vi "客户端校验.vi"() -> ()   [LabVIEW 2014]
panel:
  in  "退出":bool
  in  "生成":bool
  in  "license":string
  out "机器码":string
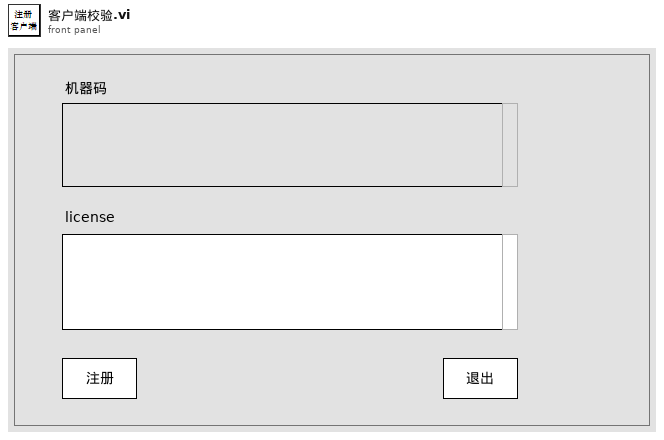
[diagram p1: front panel]
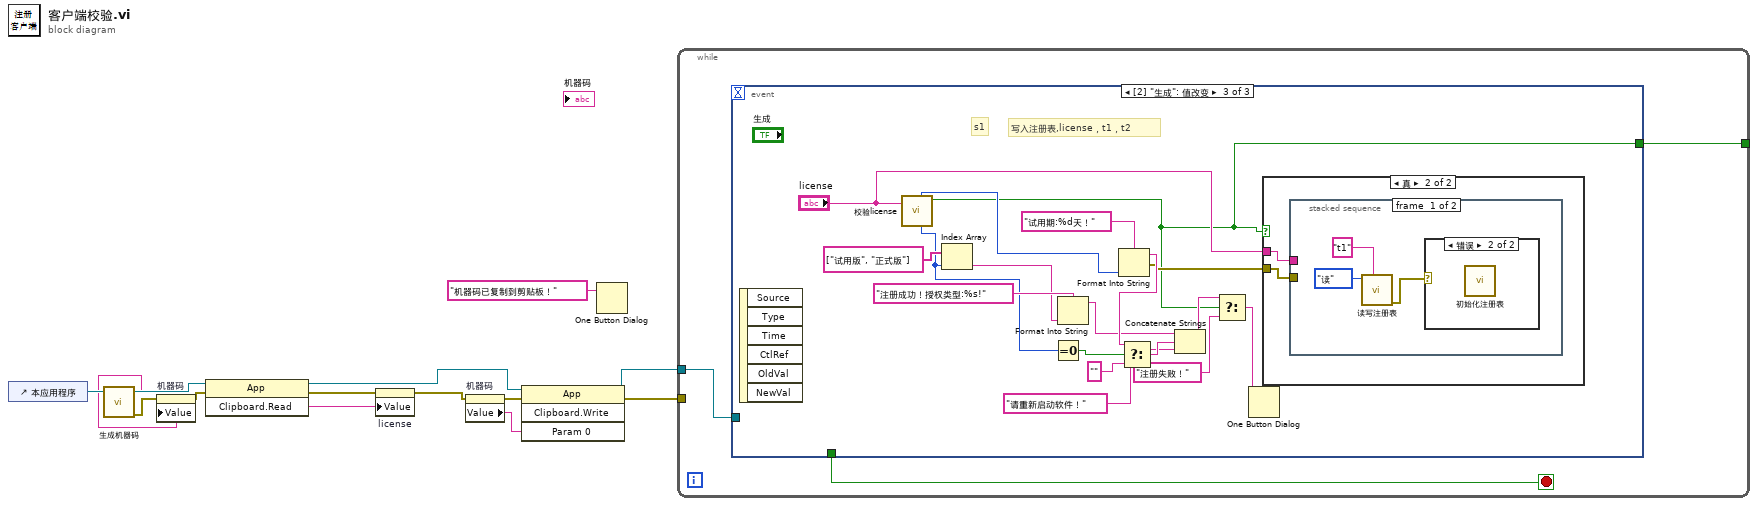
[diagram p0: block diagram]
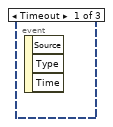
[diagram p2: hidden frame]
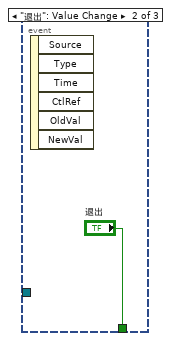
[diagram p3: hidden frame]
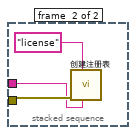
[diagram p6: hidden frame]
diagram:
  n1 = control-ref of="本应用程序"() -> (w13:refnum<vi>)
  n2 = call "生成机器码.vi"() -> ("error out"=w3:errorcluster, "机器码"=w1:string)  [unwired: 10 in]
  n3 = property on="机器码" class="Str"(error in=w3, "Value"=w1) -> (error out=w2:errorcluster)  [unwired: 1 in, 1 out]
  n4 = invoke class="App" method="Clipboard.Read"(reference=w13, error in=w2) -> (reference out=w9:refnum<vi>, error out=w12:errorcluster, "Read Clipbrd"=w11:string)  [unwired: 1 in]
  n5 = property on="license" class="Str"(error in=w12, "Value"=w11) -> (error out=w6:errorcluster)  [unwired: 1 in, 1 out]
  n6 = property on="机器码" class="Str"(error in=w6) -> (error out=w5:errorcluster, "Value"=w4:string)  [unwired: 1 in, 1 out]
  n7 = invoke class="App" method="Clipboard.Write"(reference=w9, error in=w5, "Param 0"=w4) -> (reference out=w8:refnum<vi>, error out=w7:errorcluster)  [unwired: 1 in, 2 out]
  n8 = One Button Dialog(message="机器码已复制到剪贴板！" ("消息")) -> ()  [unwired: 1 in, 1 out]
  n9 = while {
    tunnel: w8 -> [w16]
    tunnel: w7 -> [_]
    tunnel: [w14] -> _
    stop <- w15 stop-if-true
    n10 = event shown="[2] \"生成\": 值改变" {
      selector: _ -> [_ _ _]
      dyn-events: _ -> [_ _ _]
      timeout: _ -> [_ _ _]
      tunnel: w16 -> [_ _ _]
      tunnel: [_ "退出" _] -> w15
      tunnel: [_ _ w19] -> w14
      event Timeout {
        n11 = event-data() -> ()  [unwired: 1 in, 3 out]
      }
      event "退出": Value Change {
        n12 = event-data() -> ()  [unwired: 1 in, 6 out]
      }
      event "生成": Value Change {
        # "写入注册表,license，t1，t2"
        # "s1"
        n13 = event-data() -> ()  [unwired: 1 in, 6 out]
        n14 = call "校验license.vi"("license"="license") -> ("license正确"=w19:bool, "授权类型"=w30:i32, "T"=w31:u32)  [unwired: 7 in, 1 out]
        n15 = Index Array(array=string[] ["试用版", "正式版"] ("字符串[]"), index=w30) -> (element=w33:string)
        n16 = Equal To 0?(x=w30) -> (x = 0?=w29:bool)
        n17 = Format Into String(format string="注册成功！授权类型:%s!" ("格式字符串"), w33) -> (resulting string=w26:string)  [unwired: 2 in, 1 out]
        n18 = Format Into String(format string="试用期:%d天！" ("格式字符串"), w31) -> (resulting string=w28:string, error out=w21:errorcluster)  [unwired: 2 in]
        n19 = Select(t=w28, s=w29, f="") -> (s? t:f=w25:string)
        n20 = Concatenate Strings(w26, w25, "请重新启动软件！" ("字符串")) -> (w24:string)
        n21 = Select(t=w24, s=w19, f="注册失败！") -> (s? t:f=w22:string)
        n22 = One Button Dialog(message=w22) -> ()  [unwired: 1 in, 1 out]
        n23 = case shown="真" w19 {
          tunnel: w21 -> [_ w37]
          tunnel: "license" -> [_ w36]
          frame False {
          }
          frame True {
            n24 = stacked-sequence {
              tunnel: w37 -> [_ w43]
              tunnel: w36 -> [_ w41]
              frame #0 {
                n25 = call "读写注册表.vi"("键名称"="t1", "读/写"=enum16{"读", "写"}."读") -> ("error out"=w38:errorcluster)  [unwired: 8 in, 1 out]
                n26 = case shown="错误" w38 {
                  frame No Error {
                  }
                  frame Error {
                    n27 = call "初始化注册表.vi"() -> ()  [unwired: 11 in, 1 out]
                  }
                }
              }
              frame #1 {
                n28 = call "创建注册表.vi"("写入内容"=w41, "键名称"="license", "error in (no error)"=w43) -> ()  [unwired: 8 in, 1 out]
              }
            }
          }
        }
      }
    }
  }
